vi "Lab Panel V4.83.vi"() -> ()   [LabVIEW 2013] (continued)
                        n906 = TDMS Open(6:FALSE, 10:T18."create or replace" ("operation (0:open)"), 11:w1488) -> (0:w1487:errorcluster, 3:→"TDMS LAB05-2":refnum<k34>)  [unwired: 4 in]
                      }
                      frame #2 {
                        n907 = local read "SET LAB05-2"() -> (w1498:T5)
                        n908 = local read "TDMS LAB05-2"() -> (w1509:refnum<k34>)
                        n909 = Build Array("Testers Name", "Description", "Set Test Cycles", "T-Rise minutes", "T-Rise Deg C") -> (w1499:string[])
                        n910 = Unbundle(w1498) -> ("NAME"=w1497:string, "DESCRIPTION"=w1496:string, "CYCLES"=w1495:dbl, "T-RISE mins"=w1494:dbl, "T-RISE deg C"=w1493:dbl)
                        n911 = Number To Decimal String(number=w1495) -> (decimal integer string=w1508:string)  [unwired: 1 in]
                        n912 = Number To Decimal String(number=w1494) -> (decimal integer string=w1507:string)  [unwired: 1 in]
                        n913 = Number To Decimal String(number=w1493) -> (decimal integer string=w1506:string)  [unwired: 1 in]
                        n914 = Build Array(w1497, w1496, w1508, w1507, w1506) -> (w1505:string[])
                        n915 = TDMS Set Properties(5:w1505, 7:w1499, 11:w1509) -> ()  [unwired: 3 in, 4 out]
                      }
                      frame #3 {
                        w1511 = 0.0
                        n916 = local read "DISP LAB05-2"() -> (w1513:T4)
                        n917 = Bundle(cluster=w1513, "CYCLE"=w1511, "MINS"=w1511, "STATUS"="RUN") -> (w1512:T4)
                        n918 = local write "DISP LAB05-2"(w1512) -> ()
                      }
                      frame #4 {
                        n919 = local read "SIG LAB05-2"() -> (w1516:T2)
                        n920 = local read "TEMP START LAB05-2"() -> (w1518:cluster{"TL":dbl, "TN":dbl})
                        n921 = Unbundle(w1516) -> ("Tmp Live"=w1515:dbl, "Tmp Neut"=w1514:dbl)  [unwired: 3 out]
                        n922 = Bundle(cluster=w1518, "TL"=w1515, "TN"=w1514) -> (w1517:cluster{"TL":dbl, "TN":dbl})
                        n923 = local write "TEMP START LAB05-2"(w1517) -> ()
                      }
                    }
                  }
                }
              }
            }
            n924 = local write "data file error"(w580) -> ()
          }
          frame #4 {
            # "check if test cycles reached for cycle tests, if so then test pass"
            n925 = stacked-sequence {
              tunnel: w1538 -> [_ _ _ _ _ _ _ _ _ _]
              tunnel: w1537 -> [_ _ _ _ _ _ _ _ _ _]
              tunnel: w1536 -> [_ _ _ _ _ _ _ _ _ _]
              tunnel: w1535 -> [_ _ _ _ _ _ _ _ _ _]
              tunnel: w1534 -> [_ _ _ _ _ _ _ _ _ _]
              tunnel: w1533 -> [_ _ _ _ _ _ _ _ _ _]
              tunnel: w1532 -> [_ _ _ _ _ _ _ _ _ _]
              tunnel: w1531 -> [_ _ _ _ _ _ _ _ _ _]
              tunnel: w1530 -> [_ _ _ _ _ _ _ _ _ _]
              tunnel: w1529 -> [_ _ _ _ _ _ _ _ _ _]
              tunnel: w1528 -> [w1544 _ _ _ _ _ _ _ _ _]
              tunnel: w1527 -> [_ w1579 _ _ _ _ _ _ _ _]
              tunnel: w1526 -> [_ _ w1619 _ _ _ _ _ _ _]
              tunnel: w1525 -> [_ _ _ w1659 _ _ _ _ _ _]
              tunnel: w1524 -> [_ _ _ _ w1699 _ _ _ _ _]
              tunnel: w1523 -> [_ _ _ _ _ w1739 _ _ _ _]
              tunnel: w1522 -> [_ _ _ _ _ _ w1779 _ _ _]
              tunnel: w1521 -> [_ _ _ _ _ _ _ w1819 _ _]
              tunnel: w1520 -> [_ _ _ _ _ _ _ _ w1859 _]
              tunnel: w1519 -> [_ _ _ _ _ _ _ _ _ w1899]
              frame #0 {
                # "LAB01-1"
                n926 = Less?(x=w1544, y=2) -> (x < y?=w1542:bool)
                n927 = local read "DISP LAB01-1"() -> (w1545:T4)
                n928 = Unbundle(w1545) -> ("STATUS"=w1539:string)  [unwired: 2 out]
                n929 = Equal?(x=w1539, y="RUN") -> (x = y?=w1541:bool)
                n930 = And(x=w1541, y=w1542) -> (x .and. y?=w1540:bool)
                n931 = case shown="True" w1540 {
                  tunnel: w1545 -> [_ w1550]
                  tunnel: w1544 -> [_ w1554]
                  frame False {
                  }
                  frame True {
                    n932 = local read "SET LAB01-1"() -> (w1556:T5)
                    n933 = local read "TDMS LAB01-1"() -> (w1549:refnum<k34>)
                    n934 = Unbundle(w1556) -> ("CYCLES"=w1547:dbl, "T-RISE mins"=w1553:dbl)  [unwired: 3 out]
                    n935 = case shown="\"CYCLE TEST\"" w1554 {
                      tunnel: w1553 -> [_ _ w1563]
                      tunnel: [w1558 w1560 w1563] -> w1552
                      tunnel: w1547 -> [w1558 w1560 _]
                      tunnel: ["CHART PASS" "CYCLE PASS" "T-RISE PASS"] -> w1551
                      frame "CHART TEST", Default {
                      }
                      frame "CYCLE TEST" {
                      }
                      frame "T-RISE TEST" {
                      }
                    }
                    n936 = Unbundle(w1550) -> ("CYCLE"=w1555:dbl)  [unwired: 2 out]
                    n937 = Increment(x=w1547) -> (x+1=w1548:dbl)
                    n938 = Greater Or Equal?(x=w1555, y=w1548) -> (x >= y?=w1557:bool)
                    n939 = case shown="True" w1557 {
                      tunnel: w1552 -> [w1567 _]
                      tunnel: w1551 -> [w1566 _]
                      tunnel: w1550 -> [w1565 _]
                      tunnel: w1549 -> [w1564 _]
                      frame True {
                        n940 = stacked-sequence {
                          tunnel: w1567 -> [w1571 _]
                          tunnel: w1566 -> [w1569 w1575]
                          tunnel: w1565 -> [_ w1578]
                          tunnel: w1564 -> [w1568 _]
                          frame #0 {
                            n941 = Build Array(w1569) -> (w1572:string[])
                            n942 = Build Array(w1571) -> (w1570:dbl[])
                            n943 = TDMS Write(0:w1568, 5:"TEST PASS", 7:w1572, 9:w1570) -> (15:w1574:errorcluster)  [unwired: 2 in, 3 out]
                            n944 = local write "data file error"(w1574) -> ()
                          }
                          frame #1 {
                            n945 = Bundle(cluster=w1578, "STATUS"=w1575) -> (w1576:T4)  [unwired: 2 in]
                            n946 = local write "RESULT LAB01-1"(TRUE) -> ()
                            n947 = local write "DISP LAB01-1"(w1576) -> ()
                          }
                        }
                      }
                      frame False {
                      }
                    }
                  }
                }
              }
              frame #1 {
                # "LAB01-2"
                n948 = Less?(x=w1579, y=2) -> (x < y?=w1582:bool)
                n949 = local read "DISP LAB01-2"() -> (w1584:T4)
                n950 = Unbundle(w1584) -> ("STATUS"=w1585:string)  [unwired: 2 out]
                n951 = Equal?(x=w1585, y="RUN") -> (x = y?=w1581:bool)
                n952 = And(x=w1581, y=w1582) -> (x .and. y?=w1580:bool)
                n953 = case shown="True" w1580 {
                  tunnel: w1584 -> [_ w1590]
                  tunnel: w1579 -> [_ w1594]
                  frame False {
                  }
                  frame True {
                    n954 = local read "SET LAB01-2"() -> (w1596:T5)
                    n955 = local read "TDMS LAB01-2"() -> (w1589:refnum<k34>)
                    n956 = Unbundle(w1596) -> ("CYCLES"=w1587:dbl, "T-RISE mins"=w1593:dbl)  [unwired: 3 out]
                    n957 = case shown="\"T-RISE TEST\"" w1594 {
                      tunnel: w1593 -> [_ _ w1603]
                      tunnel: [w1598 w1600 w1603] -> w1592
                      tunnel: w1587 -> [w1598 w1600 _]
                      tunnel: ["CHART PASS" "CYCLE PASS" "T-RISE PASS"] -> w1591
                      frame "CHART TEST", Default {
                      }
                      frame "CYCLE TEST" {
                      }
                      frame "T-RISE TEST" {
                      }
                    }
                    n958 = Unbundle(w1590) -> ("CYCLE"=w1595:dbl)  [unwired: 2 out]
                    n959 = Increment(x=w1587) -> (x+1=w1588:dbl)
                    n960 = Greater Or Equal?(x=w1595, y=w1588) -> (x >= y?=w1597:bool)
                    n961 = case shown="True" w1597 {
                      tunnel: w1592 -> [w1607 _]
                      tunnel: w1591 -> [w1606 _]
                      tunnel: w1590 -> [w1605 _]
                      tunnel: w1589 -> [w1604 _]
                      frame True {
                        n962 = stacked-sequence {
                          tunnel: w1607 -> [w1611 _]
                          tunnel: w1606 -> [w1609 w1615]
                          tunnel: w1605 -> [_ w1618]
                          tunnel: w1604 -> [w1608 _]
                          frame #0 {
                            n963 = Build Array(w1609) -> (w1612:string[])
                            n964 = Build Array(w1611) -> (w1610:dbl[])
                            n965 = TDMS Write(0:w1608, 5:"TEST PASS", 7:w1612, 9:w1610) -> (15:w1614:errorcluster)  [unwired: 2 in, 3 out]
                            n966 = local write "data file error"(w1614) -> ()
                          }
                          frame #1 {
                            n967 = Bundle(cluster=w1618, "STATUS"=w1615) -> (w1616:T4)  [unwired: 2 in]
                            n968 = local write "RESULT LAB01-2"(TRUE) -> ()
                            n969 = local write "DISP LAB01-2"(w1616) -> ()
                          }
                        }
                      }
                      frame False {
                      }
                    }
                  }
                }
              }
              frame #2 {
                # "LAB02-1"
                n970 = Less?(x=w1619, y=2) -> (x < y?=w1622:bool)
                n971 = local read "DISP LAB02-1"() -> (w1624:T4)
                n972 = Unbundle(w1624) -> ("STATUS"=w1625:string)  [unwired: 2 out]
                n973 = Equal?(x=w1625, y="RUN") -> (x = y?=w1621:bool)
                n974 = And(x=w1621, y=w1622) -> (x .and. y?=w1620:bool)
                n975 = case shown="True" w1620 {
                  tunnel: w1624 -> [_ w1630]
                  tunnel: w1619 -> [_ w1634]
                  frame False {
                  }
                  frame True {
                    n976 = local read "SET LAB02-1"() -> (w1636:T5)
                    n977 = local read "TDMS LAB02-1"() -> (w1629:refnum<k34>)
                    n978 = Unbundle(w1630) -> ("CYCLE"=w1635:dbl)  [unwired: 2 out]
                    n979 = Unbundle(w1636) -> ("CYCLES"=w1627:dbl, "T-RISE mins"=w1633:dbl)  [unwired: 3 out]
                    n980 = case shown="\"T-RISE TEST\"" w1634 {
                      tunnel: w1633 -> [_ _ w1643]
                      tunnel: [w1638 w1640 w1643] -> w1632
                      tunnel: w1627 -> [w1638 w1640 _]
                      tunnel: ["CHART PASS" "CYCLE PASS" "T-RISE PASS"] -> w1631
                      frame "CHART TEST", Default {
                      }
                      frame "CYCLE TEST" {
                      }
                      frame "T-RISE TEST" {
                      }
                    }
                    n981 = Increment(x=w1627) -> (x+1=w1628:dbl)
                    n982 = Greater Or Equal?(x=w1635, y=w1628) -> (x >= y?=w1637:bool)
                    n983 = case shown="True" w1637 {
                      tunnel: w1632 -> [w1647 _]
                      tunnel: w1631 -> [w1646 _]
                      tunnel: w1630 -> [w1645 _]
                      tunnel: w1629 -> [w1644 _]
                      frame True {
                        n984 = stacked-sequence {
                          tunnel: w1647 -> [w1651 _]
                          tunnel: w1646 -> [w1649 w1655]
                          tunnel: w1645 -> [_ w1658]
                          tunnel: w1644 -> [w1648 _]
                          frame #0 {
                            n985 = Build Array(w1649) -> (w1652:string[])
                            n986 = Build Array(w1651) -> (w1650:dbl[])
                            n987 = TDMS Write(0:w1648, 5:"TEST PASS", 7:w1652, 9:w1650) -> (15:w1654:errorcluster)  [unwired: 2 in, 3 out]
                            n988 = local write "data file error"(w1654) -> ()
                          }
                          frame #1 {
                            n989 = Bundle(cluster=w1658, "STATUS"=w1655) -> (w1656:T4)  [unwired: 2 in]
                            n990 = local write "RESULT LAB02-1"(TRUE) -> ()
                            n991 = local write "DISP LAB02-1"(w1656) -> ()
                          }
                        }
                      }
                      frame False {
                      }
                    }
                  }
                }
              }
              frame #3 {
                # "LAB02-2"
                n992 = Less?(x=w1659, y=2) -> (x < y?=w1662:bool)
                n993 = local read "DISP LAB02-2"() -> (w1664:T4)
                n994 = Unbundle(w1664) -> ("STATUS"=w1665:string)  [unwired: 2 out]
                n995 = Equal?(x=w1665, y="RUN") -> (x = y?=w1661:bool)
                n996 = And(x=w1661, y=w1662) -> (x .and. y?=w1660:bool)
                n997 = case shown="True" w1660 {
                  tunnel: w1664 -> [_ w1670]
                  tunnel: w1659 -> [_ w1674]
                  frame False {
                  }
                  frame True {
                    n998 = local read "SET LAB02-2"() -> (w1676:T5)
                    n999 = local read "TDMS LAB02-2"() -> (w1669:refnum<k34>)
                    n1000 = Unbundle(w1670) -> ("CYCLE"=w1675:dbl)  [unwired: 2 out]
                    n1001 = Unbundle(w1676) -> ("CYCLES"=w1667:dbl, "T-RISE mins"=w1673:dbl)  [unwired: 3 out]
                    n1002 = case shown="\"T-RISE TEST\"" w1674 {
                      tunnel: w1673 -> [_ _ w1683]
                      tunnel: [w1678 w1680 w1683] -> w1672
                      tunnel: w1667 -> [w1678 w1680 _]
                      tunnel: ["CHART PASS" "CYCLE PASS" "T-RISE PASS"] -> w1671
                      frame "CHART TEST", Default {
                      }
                      frame "CYCLE TEST" {
                      }
                      frame "T-RISE TEST" {
                      }
                    }
                    n1003 = Increment(x=w1667) -> (x+1=w1668:dbl)
                    n1004 = Greater Or Equal?(x=w1675, y=w1668) -> (x >= y?=w1677:bool)
                    n1005 = case shown="True" w1677 {
                      tunnel: w1672 -> [w1687 _]
                      tunnel: w1671 -> [w1686 _]
                      tunnel: w1670 -> [w1685 _]
                      tunnel: w1669 -> [w1684 _]
                      frame True {
                        n1006 = stacked-sequence {
                          tunnel: w1687 -> [w1691 _]
                          tunnel: w1686 -> [w1689 w1695]
                          tunnel: w1685 -> [_ w1698]
                          tunnel: w1684 -> [w1688 _]
                          frame #0 {
                            n1007 = Build Array(w1689) -> (w1692:string[])
                            n1008 = Build Array(w1691) -> (w1690:dbl[])
                            n1009 = TDMS Write(0:w1688, 5:"TEST PASS", 7:w1692, 9:w1690) -> (15:w1694:errorcluster)  [unwired: 2 in, 3 out]
                            n1010 = local write "data file error"(w1694) -> ()
                          }
                          frame #1 {
                            n1011 = Bundle(cluster=w1698, "STATUS"=w1695) -> (w1696:T4)  [unwired: 2 in]
                            n1012 = local write "RESULT LAB02-2"(TRUE) -> ()
                            n1013 = local write "DISP LAB02-2"(w1696) -> ()
                          }
                        }
                      }
                      frame False {
                      }
                    }
                  }
                }
              }
              frame #4 {
                # "LAB03-1"
                n1014 = Less?(x=w1699, y=2) -> (x < y?=w1702:bool)
                n1015 = local read "DISP LAB03-1"() -> (w1704:T4)
                n1016 = Unbundle(w1704) -> ("STATUS"=w1705:string)  [unwired: 2 out]
                n1017 = Equal?(x=w1705, y="RUN") -> (x = y?=w1701:bool)
                n1018 = And(x=w1701, y=w1702) -> (x .and. y?=w1700:bool)
                n1019 = case shown="True" w1700 {
                  tunnel: w1704 -> [_ w1710]
                  tunnel: w1699 -> [_ w1714]
                  frame False {
                  }
                  frame True {
                    n1020 = local read "SET LAB03-1"() -> (w1716:T5)
                    n1021 = local read "TDMS LAB03-1"() -> (w1709:refnum<k34>)
                    n1022 = Unbundle(w1710) -> ("CYCLE"=w1715:dbl)  [unwired: 2 out]
                    n1023 = Unbundle(w1716) -> ("CYCLES"=w1707:dbl, "T-RISE mins"=w1713:dbl)  [unwired: 3 out]
                    n1024 = case shown="\"T-RISE TEST\"" w1714 {
                      tunnel: w1713 -> [_ _ w1723]
                      tunnel: [w1718 w1720 w1723] -> w1712
                      tunnel: w1707 -> [w1718 w1720 _]
                      tunnel: ["CHART PASS" "CYCLE PASS" "T-RISE PASS"] -> w1711
                      frame "CHART TEST", Default {
                      }
                      frame "CYCLE TEST" {
                      }
                      frame "T-RISE TEST" {
                      }
                    }
                    n1025 = Increment(x=w1707) -> (x+1=w1708:dbl)
                    n1026 = Greater Or Equal?(x=w1715, y=w1708) -> (x >= y?=w1717:bool)
                    n1027 = case shown="True" w1717 {
                      tunnel: w1712 -> [w1727 _]
                      tunnel: w1711 -> [w1726 _]
                      tunnel: w1710 -> [w1725 _]
                      tunnel: w1709 -> [w1724 _]
                      frame True {
                        n1028 = stacked-sequence {
                          tunnel: w1727 -> [w1731 _]
                          tunnel: w1726 -> [w1729 w1735]
                          tunnel: w1725 -> [_ w1738]
                          tunnel: w1724 -> [w1728 _]
                          frame #0 {
                            n1029 = Build Array(w1729) -> (w1732:string[])
                            n1030 = Build Array(w1731) -> (w1730:dbl[])
                            n1031 = TDMS Write(0:w1728, 5:"TEST PASS", 7:w1732, 9:w1730) -> (15:w1734:errorcluster)  [unwired: 2 in, 3 out]
                            n1032 = local write "data file error"(w1734) -> ()
                          }
                          frame #1 {
                            n1033 = Bundle(cluster=w1738, "STATUS"=w1735) -> (w1736:T4)  [unwired: 2 in]
                            n1034 = local write "RESULT LAB03-1"(TRUE) -> ()
                            n1035 = local write "DISP LAB03-1"(w1736) -> ()
                          }
                        }
                      }
                      frame False {
                      }
                    }
                  }
                }
              }
              frame #5 {
                # "LAB03-2"
                n1036 = Less?(x=w1739, y=2) -> (x < y?=w1742:bool)
                n1037 = local read "DISP LAB03-2"() -> (w1744:T4)
                n1038 = Unbundle(w1744) -> ("STATUS"=w1745:string)  [unwired: 2 out]
                n1039 = Equal?(x=w1745, y="RUN") -> (x = y?=w1741:bool)
                n1040 = And(x=w1741, y=w1742) -> (x .and. y?=w1740:bool)
                n1041 = case shown="True" w1740 {
                  tunnel: w1744 -> [_ w1750]
                  tunnel: w1739 -> [_ w1754]
                  frame False {
                  }
                  frame True {
                    n1042 = local read "SET LAB03-2"() -> (w1756:T5)
                    n1043 = local read "TDMS LAB03-2"() -> (w1749:refnum<k34>)
                    n1044 = Unbundle(w1750) -> ("CYCLE"=w1755:dbl)  [unwired: 2 out]
                    n1045 = Unbundle(w1756) -> ("CYCLES"=w1747:dbl, "T-RISE mins"=w1753:dbl)  [unwired: 3 out]
                    n1046 = case shown="\"T-RISE TEST\"" w1754 {
                      tunnel: w1753 -> [_ _ w1763]
                      tunnel: [w1758 w1760 w1763] -> w1752
                      tunnel: w1747 -> [w1758 w1760 _]
                      tunnel: ["CHART PASS" "CYCLE PASS" "T-RISE PASS"] -> w1751
                      frame "CHART TEST", Default {
                      }
                      frame "CYCLE TEST" {
                      }
                      frame "T-RISE TEST" {
                      }
                    }
                    n1047 = Increment(x=w1747) -> (x+1=w1748:dbl)
                    n1048 = Greater Or Equal?(x=w1755, y=w1748) -> (x >= y?=w1757:bool)
                    n1049 = case shown="True" w1757 {
                      tunnel: w1752 -> [w1767 _]
                      tunnel: w1751 -> [w1766 _]
                      tunnel: w1750 -> [w1765 _]
                      tunnel: w1749 -> [w1764 _]
                      frame True {
                        n1050 = stacked-sequence {
                          tunnel: w1767 -> [w1771 _]
                          tunnel: w1766 -> [w1769 w1775]
                          tunnel: w1765 -> [_ w1778]
                          tunnel: w1764 -> [w1768 _]
                          frame #0 {
                            n1051 = Build Array(w1769) -> (w1772:string[])
                            n1052 = Build Array(w1771) -> (w1770:dbl[])
                            n1053 = TDMS Write(0:w1768, 5:"TEST PASS", 7:w1772, 9:w1770) -> (15:w1774:errorcluster)  [unwired: 2 in, 3 out]
                            n1054 = local write "data file error"(w1774) -> ()
                          }
                          frame #1 {
                            n1055 = Bundle(cluster=w1778, "STATUS"=w1775) -> (w1776:T4)  [unwired: 2 in]
                            n1056 = local write "RESULT LAB03-2"(TRUE) -> ()
                            n1057 = local write "DISP LAB03-2"(w1776) -> ()
                          }
                        }
                      }
                      frame False {
                      }
                    }
                  }
                }
              }
              frame #6 {
                # "LAB04-1"
                n1058 = Less?(x=w1779, y=2) -> (x < y?=w1782:bool)
                n1059 = local read "DISP LAB04-1"() -> (w1784:T4)
                n1060 = Unbundle(w1784) -> ("STATUS"=w1785:string)  [unwired: 2 out]
                n1061 = Equal?(x=w1785, y="RUN") -> (x = y?=w1781:bool)
                n1062 = And(x=w1781, y=w1782) -> (x .and. y?=w1780:bool)
                n1063 = case shown="True" w1780 {
                  tunnel: w1784 -> [_ w1790]
                  tunnel: w1779 -> [_ w1794]
                  frame False {
                  }
                  frame True {
                    n1064 = local read "SET LAB04-1"() -> (w1796:T5)
                    n1065 = local read "TDMS LAB04-1"() -> (w1789:refnum<k34>)
                    n1066 = Unbundle(w1790) -> ("CYCLE"=w1795:dbl)  [unwired: 2 out]
                    n1067 = Unbundle(w1796) -> ("CYCLES"=w1787:dbl, "T-RISE mins"=w1793:dbl)  [unwired: 3 out]
                    n1068 = case shown="\"T-RISE TEST\"" w1794 {
                      tunnel: w1793 -> [_ _ w1803]
                      tunnel: [w1798 w1800 w1803] -> w1792
                      tunnel: w1787 -> [w1798 w1800 _]
                      tunnel: ["CHART PASS" "CYCLE PASS" "T-RISE PASS"] -> w1791
                      frame "CHART TEST", Default {
                      }
                      frame "CYCLE TEST" {
                      }
                      frame "T-RISE TEST" {
                      }
                    }
                    n1069 = Increment(x=w1787) -> (x+1=w1788:dbl)
                    n1070 = Greater Or Equal?(x=w1795, y=w1788) -> (x >= y?=w1797:bool)
                    n1071 = case shown="True" w1797 {
                      tunnel: w1792 -> [w1807 _]
                      tunnel: w1791 -> [w1806 _]
                      tunnel: w1790 -> [w1805 _]
                      tunnel: w1789 -> [w1804 _]
                      frame True {
                        n1072 = stacked-sequence {
                          tunnel: w1807 -> [w1811 _]
                          tunnel: w1806 -> [w1809 w1815]
                          tunnel: w1805 -> [_ w1818]
                          tunnel: w1804 -> [w1808 _]
                          frame #0 {
                            n1073 = Build Array(w1809) -> (w1812:string[])
                            n1074 = Build Array(w1811) -> (w1810:dbl[])
                            n1075 = TDMS Write(0:w1808, 5:"TEST PASS", 7:w1812, 9:w1810) -> (15:w1814:errorcluster)  [unwired: 2 in, 3 out]
                            n1076 = local write "data file error"(w1814) -> ()
                          }
                          frame #1 {
                            n1077 = Bundle(cluster=w1818, "STATUS"=w1815) -> (w1816:T4)  [unwired: 2 in]
                            n1078 = local write "RESULT LAB04-1"(TRUE) -> ()
                            n1079 = local write "DISP LAB04-1"(w1816) -> ()
                          }
                        }
                      }
                      frame False {
                      }
                    }
                  }
                }
              }
              frame #7 {
                # "LAB04-2"
                n1080 = Less?(x=w1819, y=2) -> (x < y?=w1822:bool)
                n1081 = local read "DISP LAB04-2"() -> (w1824:T4)
                n1082 = Unbundle(w1824) -> ("STATUS"=w1825:string)  [unwired: 2 out]
                n1083 = Equal?(x=w1825, y="RUN") -> (x = y?=w1821:bool)
                n1084 = And(x=w1821, y=w1822) -> (x .and. y?=w1820:bool)
                n1085 = case shown="True" w1820 {
                  tunnel: w1824 -> [_ w1830]
                  tunnel: w1819 -> [_ w1834]
                  frame False {
                  }
                  frame True {
                    n1086 = local read "SET LAB04-2"() -> (w1836:T5)
                    n1087 = local read "TDMS LAB04-2"() -> (w1829:refnum<k34>)
                    n1088 = Unbundle(w1830) -> ("CYCLE"=w1835:dbl)  [unwired: 2 out]
                    n1089 = Unbundle(w1836) -> ("CYCLES"=w1827:dbl, "T-RISE mins"=w1833:dbl)  [unwired: 3 out]
                    n1090 = case shown="\"T-RISE TEST\"" w1834 {
                      tunnel: w1833 -> [_ _ w1843]
                      tunnel: [w1838 w1840 w1843] -> w1832
                      tunnel: w1827 -> [w1838 w1840 _]
                      tunnel: ["CHART PASS" "CYCLE PASS" "T-RISE PASS"] -> w1831
                      frame "CHART TEST", Default {
                      }
                      frame "CYCLE TEST" {
                      }
                      frame "T-RISE TEST" {
                      }
                    }
                    n1091 = Increment(x=w1827) -> (x+1=w1828:dbl)
                    n1092 = Greater Or Equal?(x=w1835, y=w1828) -> (x >= y?=w1837:bool)
                    n1093 = case shown="True" w1837 {
                      tunnel: w1832 -> [w1847 _]
                      tunnel: w1831 -> [w1846 _]
                      tunnel: w1830 -> [w1845 _]
                      tunnel: w1829 -> [w1844 _]
                      frame True {
                        n1094 = stacked-sequence {
                          tunnel: w1847 -> [w1851 _]
                          tunnel: w1846 -> [w1849 w1855]
                          tunnel: w1845 -> [_ w1858]
                          tunnel: w1844 -> [w1848 _]
                          frame #0 {
                            n1095 = Build Array(w1849) -> (w1852:string[])
                            n1096 = Build Array(w1851) -> (w1850:dbl[])
                            n1097 = TDMS Write(0:w1848, 5:"TEST PASS", 7:w1852, 9:w1850) -> (15:w1854:errorcluster)  [unwired: 2 in, 3 out]
                            n1098 = local write "data file error"(w1854) -> ()
                          }
                          frame #1 {
                            n1099 = Bundle(cluster=w1858, "STATUS"=w1855) -> (w1856:T4)  [unwired: 2 in]
                            n1100 = local write "RESULT LAB04-2"(TRUE) -> ()
                            n1101 = local write "DISP LAB04-2"(w1856) -> ()
                          }
                        }
                      }
                      frame False {
                      }
                    }
                  }
                }
              }
              frame #8 {
                # "LAB05-1"
                n1102 = Less?(x=w1859, y=2) -> (x < y?=w1862:bool)
                n1103 = local read "DISP LAB05-1"() -> (w1864:T4)
                n1104 = Unbundle(w1864) -> ("STATUS"=w1865:string)  [unwired: 2 out]
                n1105 = Equal?(x=w1865, y="RUN") -> (x = y?=w1861:bool)
                n1106 = And(x=w1861, y=w1862) -> (x .and. y?=w1860:bool)
                n1107 = case shown="True" w1860 {
                  tunnel: w1864 -> [_ w1870]
                  tunnel: w1859 -> [_ w1874]
                  frame False {
                  }
                  frame True {
                    n1108 = local read "SET LAB05-1"() -> (w1876:T5)
                    n1109 = local read "TDMS LAB05-1"() -> (w1869:refnum<k34>)
                    n1110 = Unbundle(w1870) -> ("CYCLE"=w1875:dbl)  [unwired: 2 out]
                    n1111 = Unbundle(w1876) -> ("CYCLES"=w1867:dbl, "T-RISE mins"=w1873:dbl)  [unwired: 3 out]
                    n1112 = case shown="\"T-RISE TEST\"" w1874 {
                      tunnel: w1873 -> [_ _ w1883]
                      tunnel: [w1878 w1880 w1883] -> w1872
                      tunnel: w1867 -> [w1878 w1880 _]
                      tunnel: ["CHART PASS" "CYCLE PASS" "T-RISE PASS"] -> w1871
                      frame "CHART TEST", Default {
                      }
                      frame "CYCLE TEST" {
                      }
                      frame "T-RISE TEST" {
                      }
                    }
                    n1113 = Increment(x=w1867) -> (x+1=w1868:dbl)
                    n1114 = Greater Or Equal?(x=w1875, y=w1868) -> (x >= y?=w1877:bool)
                    n1115 = case shown="True" w1877 {
                      tunnel: w1872 -> [w1887 _]
                      tunnel: w1871 -> [w1886 _]
                      tunnel: w1870 -> [w1885 _]
                      tunnel: w1869 -> [w1884 _]
                      frame True {
                        n1116 = stacked-sequence {
                          tunnel: w1887 -> [w1891 _]
                          tunnel: w1886 -> [w1889 w1895]
                          tunnel: w1885 -> [_ w1898]
                          tunnel: w1884 -> [w1888 _]
                          frame #0 {
                            n1117 = Build Array(w1889) -> (w1892:string[])
                            n1118 = Build Array(w1891) -> (w1890:dbl[])
                            n1119 = TDMS Write(0:w1888, 5:"TEST PASS", 7:w1892, 9:w1890) -> (15:w1894:errorcluster)  [unwired: 2 in, 3 out]
                            n1120 = local write "data file error"(w1894) -> ()
                          }
                          frame #1 {
                            n1121 = Bundle(cluster=w1898, "STATUS"=w1895) -> (w1896:T4)  [unwired: 2 in]
                            n1122 = local write "RESULT LAB05-1"(TRUE) -> ()
                            n1123 = local write "DISP LAB05-1"(w1896) -> ()
                          }
                        }
                      }
                      frame False {
                      }
                    }
                  }
                }
              }
              frame #9 {
                # "LAB05-2"
                n1124 = Less?(x=w1899, y=2) -> (x < y?=w1902:bool)
                n1125 = local read "DISP LAB05-2"() -> (w1904:T4)
                n1126 = Unbundle(w1904) -> ("STATUS"=w1905:string)  [unwired: 2 out]
                n1127 = Equal?(x=w1905, y="RUN") -> (x = y?=w1901:bool)
                n1128 = And(x=w1901, y=w1902) -> (x .and. y?=w1900:bool)
                n1129 = case shown="True" w1900 {
                  tunnel: w1904 -> [_ w1910]
                  tunnel: w1899 -> [_ w1914]
                  frame False {
                  }
                  frame True {
                    n1130 = local read "SET LAB05-2"() -> (w1916:T5)
                    n1131 = local read "TDMS LAB05-2"() -> (w1909:refnum<k34>)
                    n1132 = Unbundle(w1910) -> ("CYCLE"=w1915:dbl)  [unwired: 2 out]
                    n1133 = Unbundle(w1916) -> ("CYCLES"=w1907:dbl, "T-RISE mins"=w1913:dbl)  [unwired: 3 out]
                    n1134 = case shown="\"T-RISE TEST\"" w1914 {
                      tunnel: w1913 -> [_ _ w1923]
                      tunnel: [w1918 w1920 w1923] -> w1912
                      tunnel: w1907 -> [w1918 w1920 _]
                      tunnel: ["CHART PASS" "CYCLE PASS" "T-RISE PASS"] -> w1911
                      frame "CHART TEST", Default {
                      }
                      frame "CYCLE TEST" {
                      }
                      frame "T-RISE TEST" {
                      }
                    }
                    n1135 = Increment(x=w1907) -> (x+1=w1908:dbl)
                    n1136 = Greater Or Equal?(x=w1915, y=w1908) -> (x >= y?=w1917:bool)
                    n1137 = case shown="True" w1917 {
                      tunnel: w1912 -> [w1927 _]
                      tunnel: w1911 -> [w1926 _]
                      tunnel: w1910 -> [w1925 _]
                      tunnel: w1909 -> [w1924 _]
                      frame True {
                        n1138 = stacked-sequence {
                          tunnel: w1927 -> [w1931 _]
                          tunnel: w1926 -> [w1929 w1935]
                          tunnel: w1925 -> [_ w1938]
                          tunnel: w1924 -> [w1928 _]
                          frame #0 {
                            n1139 = Build Array(w1929) -> (w1932:string[])
                            n1140 = Build Array(w1931) -> (w1930:dbl[])
                            n1141 = TDMS Write(0:w1928, 5:"TEST PASS", 7:w1932, 9:w1930) -> (15:w1934:errorcluster)  [unwired: 2 in, 3 out]
                            n1142 = local write "data file error"(w1934) -> ()
                          }
                          frame #1 {
                            n1143 = Bundle(cluster=w1938, "STATUS"=w1935) -> (w1936:T4)  [unwired: 2 in]
                            n1144 = local write "RESULT LAB05-2"(TRUE) -> ()
                            n1145 = local write "DISP LAB05-2"(w1936) -> ()
                          }
                        }
                      }
                      frame False {
                      }
                    }
                  }
                }
              }
            }
          }
          frame #5 {
            # "check if test cycles reached for temperature rise test"
            n1146 = stacked-sequence {
              tunnel: w1968 -> [_ _ _ _ _ _ _ _ _ _]
              tunnel: w1967 -> [_ _ _ _ _ _ _ _ _ _]
              tunnel: w1966 -> [_ _ _ _ _ _ _ _ _ _]
              tunnel: w1965 -> [_ _ _ _ _ _ _ _ _ _]
              tunnel: w1964 -> [_ _ _ _ _ _ _ _ _ _]
              tunnel: w1963 -> [_ _ _ _ _ _ _ _ _ _]
              tunnel: w1962 -> [_ _ _ _ _ _ _ _ _ _]
              tunnel: w1961 -> [_ _ _ _ _ _ _ _ _ _]
              tunnel: w1960 -> [_ _ _ _ _ _ _ _ _ _]
              tunnel: w1959 -> [_ _ _ _ _ _ _ _ _ _]
              tunnel: w1958 -> [w1974 _ _ _ _ _ _ _ _ _]
              tunnel: w1948 -> [w1969 _ _ _ _ _ _ _ _ _]
              tunnel: w1957 -> [_ w2000 _ _ _ _ _ _ _ _]
              tunnel: w1956 -> [_ _ w2030 _ _ _ _ _ _ _]
              tunnel: w1955 -> [_ _ _ w2060 _ _ _ _ _ _]
              tunnel: w1954 -> [_ _ _ _ w2090 _ _ _ _ _]
              tunnel: w1953 -> [_ _ _ _ _ w2120 _ _ _ _]
              tunnel: w1952 -> [_ _ _ _ _ _ w2150 _ _ _]
              tunnel: w1951 -> [_ _ _ _ _ _ _ w2180 _ _]
              tunnel: w1950 -> [_ _ _ _ _ _ _ _ w2210 _]
              tunnel: w1949 -> [_ _ _ _ _ _ _ _ _ w2240]
              tunnel: w1947 -> [_ w1999 _ _ _ _ _ _ _ _]
              tunnel: w1946 -> [_ _ w2029 _ _ _ _ _ _ _]
              tunnel: w1945 -> [_ _ _ w2059 _ _ _ _ _ _]
              tunnel: w1944 -> [_ _ _ _ w2089 _ _ _ _ _]
              tunnel: w1943 -> [_ _ _ _ _ w2119 _ _ _ _]
              tunnel: w1942 -> [_ _ _ _ _ _ w2149 _ _ _]
              tunnel: w1941 -> [_ _ _ _ _ _ _ w2179 _ _]
              tunnel: w1940 -> [_ _ _ _ _ _ _ _ w2209 _]
              tunnel: w1939 -> [_ _ _ _ _ _ _ _ _ w2239]
              frame #0 {
                # "LAB01-1"
                n1147 = Equal?(x=w1974, y=2) -> (x = y?=w1972:bool)
                n1148 = local read "DISP LAB01-1"() -> (w1975:T4)
                n1149 = Unbundle(w1975) -> ("STATUS"=w1976:string)  [unwired: 2 out]
                n1150 = Equal?(x=w1976, y="RUN") -> (x = y?=w1971:bool)
                n1151 = And(x=w1971, y=w1972) -> (x .and. y?=w1970:bool)
                n1152 = case shown="True" w1970 {
                  tunnel: w1975 -> [_ w1979]
                  tunnel: w1969 -> [_ w1982]
                  frame False {
                  }
                  frame True {
                    n1153 = local read "SET LAB01-1"() -> (w1981:T5)
                    n1154 = local read "TDMS LAB01-1"() -> (w1978:refnum<k34>)
                    n1155 = Unbundle(w1979) -> ("CYCLE"=w1983:dbl)  [unwired: 2 out]
                    n1156 = Unbundle(w1981) -> ("T-RISE mins"=w1980:dbl)  [unwired: 4 out]
                    n1157 = Greater Or Equal?(x=w1983, y=w1982) -> (x >= y?=w1984:bool)
                    n1158 = case shown="True" w1984 {
                      tunnel: w1980 -> [w1987 _]
                      tunnel: w1979 -> [w1986 _]
                      tunnel: w1978 -> [w1985 _]
                      frame True {
                        n1159 = stacked-sequence {
                          tunnel: w1987 -> [w1990 _]
                          tunnel: w1986 -> [_ w1995]
                          tunnel: w1985 -> [w1988 _]
                          frame #0 {
                            n1160 = Build Array("T-RISE") -> (w1992:string[])
                            n1161 = Build Array(w1990) -> (w1991:dbl[])
                            n1162 = TDMS Write(0:w1988, 5:"TEST PASS", 7:w1992, 9:w1991) -> (15:w1994:errorcluster)  [unwired: 2 in, 3 out]
                            n1163 = local write "data file error"(w1994) -> ()
                          }
                          frame #1 {
                            n1164 = Bundle(cluster=w1995, "STATUS"="T-RISE PASS") -> (w1997:T4)  [unwired: 2 in]
                            n1165 = local write "RESULT LAB01-1"(TRUE) -> ()
                            n1166 = local write "DISP LAB01-1"(w1997) -> ()
                          }
                        }
                      }
                      frame False {
                      }
                    }
                  }
                }
              }
              frame #1 {
                # "LAB01-2"
                n1167 = Equal?(x=w2000, y=2) -> (x = y?=w2003:bool)
                n1168 = local read "DISP LAB01-2"() -> (w2005:T4)
                n1169 = Unbundle(w2005) -> ("STATUS"=w2006:string)  [unwired: 2 out]
                n1170 = Equal?(x=w2006, y="RUN") -> (x = y?=w2002:bool)
                n1171 = And(x=w2002, y=w2003) -> (x .and. y?=w2001:bool)
                n1172 = case shown="True" w2001 {
                  tunnel: w2005 -> [_ w2009]
                  tunnel: w1999 -> [_ w2012]
                  frame False {
                  }
                  frame True {
                    n1173 = local read "SET LAB01-2"() -> (w2011:T5)
                    n1174 = local read "TDMS LAB01-2"() -> (w2008:refnum<k34>)
                    n1175 = Unbundle(w2009) -> ("CYCLE"=w2013:dbl)  [unwired: 2 out]
                    n1176 = Unbundle(w2011) -> ("T-RISE mins"=w2010:dbl)  [unwired: 4 out]
                    n1177 = Greater Or Equal?(x=w2013, y=w2012) -> (x >= y?=w2014:bool)
                    n1178 = case shown="True" w2014 {
                      tunnel: w2010 -> [w2017 _]
                      tunnel: w2009 -> [w2016 _]
                      tunnel: w2008 -> [w2015 _]
                      frame True {
                        n1179 = stacked-sequence {
                          tunnel: w2017 -> [w2020 _]
                          tunnel: w2016 -> [_ w2025]
                          tunnel: w2015 -> [w2018 _]
                          frame #0 {
                            n1180 = Build Array("T-RISE") -> (w2022:string[])
                            n1181 = Build Array(w2020) -> (w2021:dbl[])
                            n1182 = TDMS Write(0:w2018, 5:"TEST PASS", 7:w2022, 9:w2021) -> (15:w2024:errorcluster)  [unwired: 2 in, 3 out]
                            n1183 = local write "data file error"(w2024) -> ()
                          }
                          frame #1 {
                            n1184 = Bundle(cluster=w2025, "STATUS"="T-RISE PASS") -> (w2027:T4)  [unwired: 2 in]
                            n1185 = local write "RESULT LAB01-2"(TRUE) -> ()
                            n1186 = local write "DISP LAB01-2"(w2027) -> ()
                          }
                        }
                      }
                      frame False {
                      }
                    }
                  }
                }
              }
              frame #2 {
                # "LAB02-1"
                n1187 = Equal?(x=w2030, y=2) -> (x = y?=w2033:bool)
                n1188 = local read "DISP LAB02-1"() -> (w2035:T4)
                n1189 = Unbundle(w2035) -> ("STATUS"=w2036:string)  [unwired: 2 out]
                n1190 = Equal?(x=w2036, y="RUN") -> (x = y?=w2032:bool)
                n1191 = And(x=w2032, y=w2033) -> (x .and. y?=w2031:bool)
                n1192 = case shown="True" w2031 {
                  tunnel: w2035 -> [_ w2039]
                  tunnel: w2029 -> [_ w2042]
                  frame False {
                  }
                  frame True {
                    n1193 = local read "SET LAB02-1"() -> (w2041:T5)
                    n1194 = local read "TDMS LAB02-1"() -> (w2038:refnum<k34>)
                    n1195 = Unbundle(w2039) -> ("CYCLE"=w2043:dbl)  [unwired: 2 out]
                    n1196 = Unbundle(w2041) -> ("T-RISE mins"=w2040:dbl)  [unwired: 4 out]
                    n1197 = Greater Or Equal?(x=w2043, y=w2042) -> (x >= y?=w2044:bool)
                    n1198 = case shown="True" w2044 {
                      tunnel: w2040 -> [w2047 _]
                      tunnel: w2039 -> [w2046 _]
                      tunnel: w2038 -> [w2045 _]
                      frame True {
                        n1199 = stacked-sequence {
                          tunnel: w2047 -> [w2050 _]
                          tunnel: w2046 -> [_ w2055]
                          tunnel: w2045 -> [w2048 _]
                          frame #0 {
                            n1200 = Build Array("T-RISE") -> (w2052:string[])
                            n1201 = Build Array(w2050) -> (w2051:dbl[])
                            n1202 = TDMS Write(0:w2048, 5:"TEST PASS", 7:w2052, 9:w2051) -> (15:w2054:errorcluster)  [unwired: 2 in, 3 out]
                            n1203 = local write "data file error"(w2054) -> ()
                          }
                          frame #1 {
                            n1204 = Bundle(cluster=w2055, "STATUS"="T-RISE PASS") -> (w2057:T4)  [unwired: 2 in]
                            n1205 = local write "RESULT LAB02-1"(TRUE) -> ()
                            n1206 = local write "DISP LAB02-1"(w2057) -> ()
                          }
                        }
                      }
                      frame False {
                      }
                    }
                  }
                }
              }
              frame #3 {
                # "LAB02-2"
                n1207 = Equal?(x=w2060, y=2) -> (x = y?=w2063:bool)
                n1208 = local read "DISP LAB02-2"() -> (w2065:T4)
                n1209 = Unbundle(w2065) -> ("STATUS"=w2066:string)  [unwired: 2 out]
                n1210 = Equal?(x=w2066, y="RUN") -> (x = y?=w2062:bool)
                n1211 = And(x=w2062, y=w2063) -> (x .and. y?=w2061:bool)
                n1212 = case shown="True" w2061 {
                  tunnel: w2065 -> [_ w2069]
                  tunnel: w2059 -> [_ w2072]
                  frame False {
                  }
                  frame True {
                    n1213 = local read "SET LAB02-2"() -> (w2071:T5)
                    n1214 = local read "TDMS LAB02-2"() -> (w2068:refnum<k34>)
                    n1215 = Unbundle(w2069) -> ("CYCLE"=w2073:dbl)  [unwired: 2 out]
                    n1216 = Unbundle(w2071) -> ("T-RISE mins"=w2070:dbl)  [unwired: 4 out]
                    n1217 = Greater Or Equal?(x=w2073, y=w2072) -> (x >= y?=w2074:bool)
                    n1218 = case shown="True" w2074 {
                      tunnel: w2070 -> [w2077 _]
                      tunnel: w2069 -> [w2076 _]
                      tunnel: w2068 -> [w2075 _]
                      frame True {
                        n1219 = stacked-sequence {
                          tunnel: w2077 -> [w2080 _]
                          tunnel: w2076 -> [_ w2085]
                          tunnel: w2075 -> [w2078 _]
                          frame #0 {
                            n1220 = Build Array("T-RISE") -> (w2082:string[])
                            n1221 = Build Array(w2080) -> (w2081:dbl[])
                            n1222 = TDMS Write(0:w2078, 5:"TEST PASS", 7:w2082, 9:w2081) -> (15:w2084:errorcluster)  [unwired: 2 in, 3 out]
                            n1223 = local write "data file error"(w2084) -> ()
                          }
                          frame #1 {
                            n1224 = Bundle(cluster=w2085, "STATUS"="T-RISE PASS") -> (w2087:T4)  [unwired: 2 in]
                            n1225 = local write "RESULT LAB02-2"(TRUE) -> ()
                            n1226 = local write "DISP LAB02-2"(w2087) -> ()
                          }
                        }
                      }
                      frame False {
                      }
                    }
                  }
                }
              }
              frame #4 {
                # "LAB03-1"
                n1227 = Equal?(x=w2090, y=2) -> (x = y?=w2093:bool)
                n1228 = local read "DISP LAB03-1"() -> (w2095:T4)
                n1229 = Unbundle(w2095) -> ("STATUS"=w2096:string)  [unwired: 2 out]
                n1230 = Equal?(x=w2096, y="RUN") -> (x = y?=w2092:bool)
                n1231 = And(x=w2092, y=w2093) -> (x .and. y?=w2091:bool)
                n1232 = case shown="True" w2091 {
                  tunnel: w2095 -> [_ w2099]
                  tunnel: w2089 -> [_ w2102]
                  frame False {
                  }
                  frame True {
                    n1233 = local read "SET LAB03-1"() -> (w2101:T5)
                    n1234 = local read "TDMS LAB03-1"() -> (w2098:refnum<k34>)
                    n1235 = Unbundle(w2099) -> ("CYCLE"=w2103:dbl)  [unwired: 2 out]
                    n1236 = Unbundle(w2101) -> ("T-RISE mins"=w2100:dbl)  [unwired: 4 out]
                    n1237 = Greater Or Equal?(x=w2103, y=w2102) -> (x >= y?=w2104:bool)
                    n1238 = case shown="True" w2104 {
                      tunnel: w2100 -> [w2107 _]
                      tunnel: w2099 -> [w2106 _]
                      tunnel: w2098 -> [w2105 _]
                      frame True {
                        n1239 = stacked-sequence {
                          tunnel: w2107 -> [w2110 _]
                          tunnel: w2106 -> [_ w2115]
                          tunnel: w2105 -> [w2108 _]
                          frame #0 {
                            n1240 = Build Array("T-RISE") -> (w2112:string[])
                            n1241 = Build Array(w2110) -> (w2111:dbl[])
                            n1242 = TDMS Write(0:w2108, 5:"TEST PASS", 7:w2112, 9:w2111) -> (15:w2114:errorcluster)  [unwired: 2 in, 3 out]
